vi "Remanent Magnetization Callculate.vi"(10 "H":dbl[](array[numeric]), 11 "B":dbl[](array[numeric])) -> (1 "Br":dbl, 2 "Downward":dbl, 3 "Upward":dbl)   [LabVIEW 2019]
uses:
  <vilib>/gmath/NI_Gmath.lvlib
panel:
  out "array size":i32
  out "x 1":dbl[](array[numeric])
  out "y1":dbl[](array[numeric])
  out "x2":dbl[](array[numeric])
  out "y2":dbl[](array[numeric])
  out "XY Graph":cluster{"data":dbl[], "data":dbl[]}(graph)
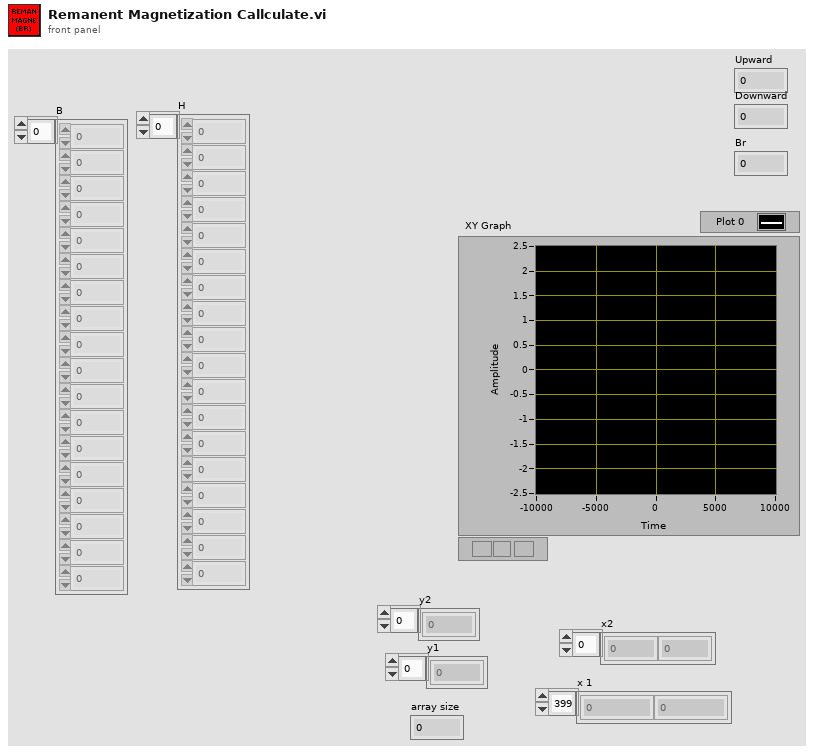
[diagram p1: front panel]
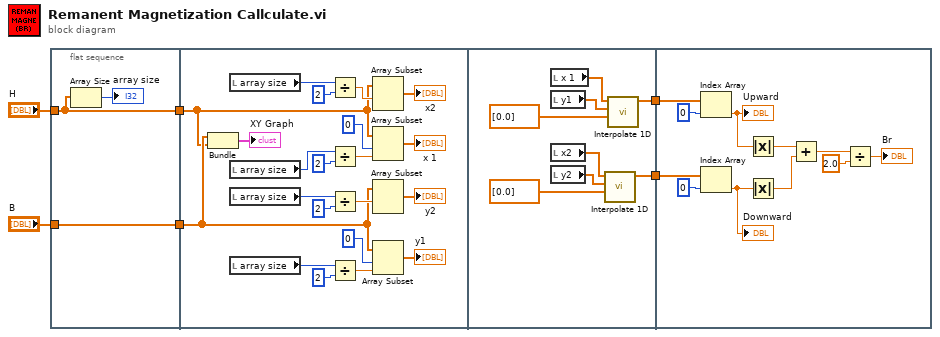
[diagram p0: block diagram]
diagram:
  n1 = flat-sequence {
    tunnel: "H" -> [w7]
    tunnel: "B" -> [w9]
    tunnel: [w9] -> w2
    tunnel: [w7] -> w1
    tunnel: w2 -> [w11]
    tunnel: w1 -> [w10]
    tunnel: [w32] -> w4
    tunnel: [w31] -> w3
    tunnel: w4 -> [w41]
    tunnel: w3 -> [w40]
    frame #0 {
      n2 = Array Size(array=w7) -> (size(s)=→"array size":i32)
    }
    frame #1 {
      n3 = Bundle("B"=w11, "H"=w10) -> (→"XY Graph":cluster{"B":dbl[], "H":dbl[]})  [unwired: 1 in]
      n4 = local read "array size"() -> (w22:i32)
      n5 = local read "array size"() -> (w14:i32)
      n6 = local read "array size"() -> (w27:i32)
      n7 = local read "array size"() -> (w19:i32)
      n8 = Divide(x=w22, y=2) -> (x/y=w24:dbl)
      n9 = Divide(x=w14, y=2) -> (x/y=w16:dbl)
      n10 = Divide(x=w27, y=2) -> (x/y=w25:dbl)
      n11 = Divide(x=w19, y=2) -> (x/y=w17:dbl)
      n12 = Array Subset(array=w10, index=w24) -> (→"x2":dbl[])  [unwired: 1 in]
      n13 = Array Subset(array=w10, index=0, length=w16) -> (→"x 1":dbl[])
      n14 = Array Subset(array=w11, index=w25) -> (→"y2":dbl[])  [unwired: 1 in]
      n15 = Array Subset(array=w11, index=0, length=w17) -> (→"y1":dbl[])
    }
    frame #2 {
      n16 = local read "x 1"() -> (w35:dbl[])
      n17 = local read "y1"() -> (w36:dbl[])
      n18 = local read "x2"() -> (w34:dbl[])
      n19 = local read "y2"() -> (w33:dbl[])
      n20 = call <vilib>:"Interpolate 1D.vi"("xi"=dbl[] [0.0], "X"=w33, "Y"=w34) -> ("yi"=w31:dbl[])  [unwired: 6 in, 2 out]
      n21 = call <vilib>:"Interpolate 1D.vi"("xi"=dbl[] [0.0], "X"=w36, "Y"=w35) -> ("yi"=w32:dbl[])  [unwired: 6 in, 2 out]
    }
    frame #3 {
      n22 = Index Array(array=w41, index=0) -> (element=w47:dbl)
      "Upward" <- w47
      n23 = Index Array(array=w40, index=0) -> (element=w39:dbl)
      "Downward" <- w39
      n24 = Absolute Value(x=w47) -> (abs(x)=w46:dbl)
      n25 = Absolute Value(x=w39) -> (abs(x)=w45:dbl)
      n26 = Add(x=w46, y=w45) -> (x+y=w44:dbl)
      n27 = Divide(x=w44, y=2.0) -> (x/y=→"Br":dbl)
    }
  }
